vi "host.vi"() -> ()   [LabVIEW 2020]
uses:
  <vilib>/rvi/interface/nirviOpenFPGA/nirviOpenFPGA.xnode
  <vilib>/rvi/interface/nirviCloseFPGA/nirviCloseFPGA.xnode
  <vilib>/rvi/interface/nirviMethod/nirviMethod.xnode
  <vilib>/FPGAPlugInAG/Dynamic/niLvFpga_Run_Dynamic.vi
  <vilib>/rvi/errors/niLvFpgaMergeErrorWithErrorCode.vi
  <vilib>/Analysis/NI_AALBase.lvlib
  <vilib>/Analysis/baseanly.llb/Real A x B.vi
  <vilib>/Analysis/baseanly.llb/Mean (DBL).vi
  <vilib>/Analysis/NI_AALPro.lvlib
  <vilib>/Analysis/7linalg.llb/Real Cholesky Factorization.vi
  <vilib>/Analysis/7linalg.llb/Real Transpose Matrix.vi
  <vilib>/Analysis/baseanly.llb/Real Inverse Matrix.vi
  <vilib>/Analysis/7linalg.llb/Real Eigenvalues and Vectors.vi
  <vilib>/rvi/interface/nirviReadWriteControl/nirviReadWriteControl.xnode
  <vilib>/FPGAPlugInAG/Dynamic/niLvFpga_WriteFifo_Dynamic.vi
  NiFpgaLv.dll
  <vilib>/Utility/error.llb/Error Cluster From Error Code.vi
  <vilib>/rvi/interface/Simulation/niFpgaSimulationCallBeginRW.vi
  <vilib>/rvi/errors/niLvFpgaAdjustHostInterfaceError.vi
  <vilib>/FPGAPlugInAG/Dynamic/niLvFpga_ReadFifo_Dynamic.vi
  <vilib>/FPGAPlugInAG/Dynamic/niLvFpga_Close_Dynamic.vi
  FPGA Bitfiles/labviewfpgacheck_FPGATarget2_target_3W1cPbM74FU.lvbitx
  target.vi
  <vilib>/FPGAPlugInAG/PXIe-5763 (KU060)/niLvFpga_Open_PXIe-5763 (KU060).vi
  <vilib>/rvi/interface/common/dynamic/niFpgaDynamicAddResources.vi
panel:
  out "time (ms)":dbl
  out "tick count":u32
  out "LabVIEW eigvals":dbl[](array[numeric])
  out "FPGA Jacobi eigenvalue":sgl[](array[numeric])
  out "percent error":dbl
  out "A":sgl[][](array[numeric])
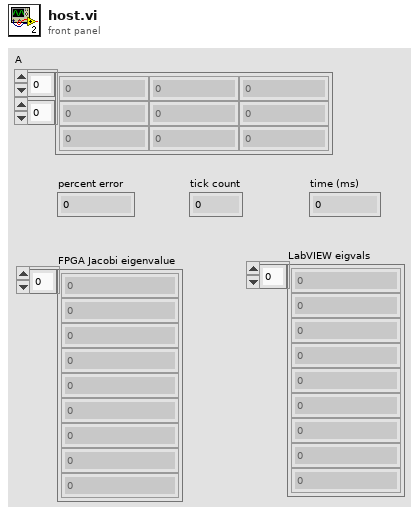
[diagram p1: front panel]
types:
  T1 = typedef "NI_Matrix.lvlib/RealMatrix.ctl" = dbl[][]
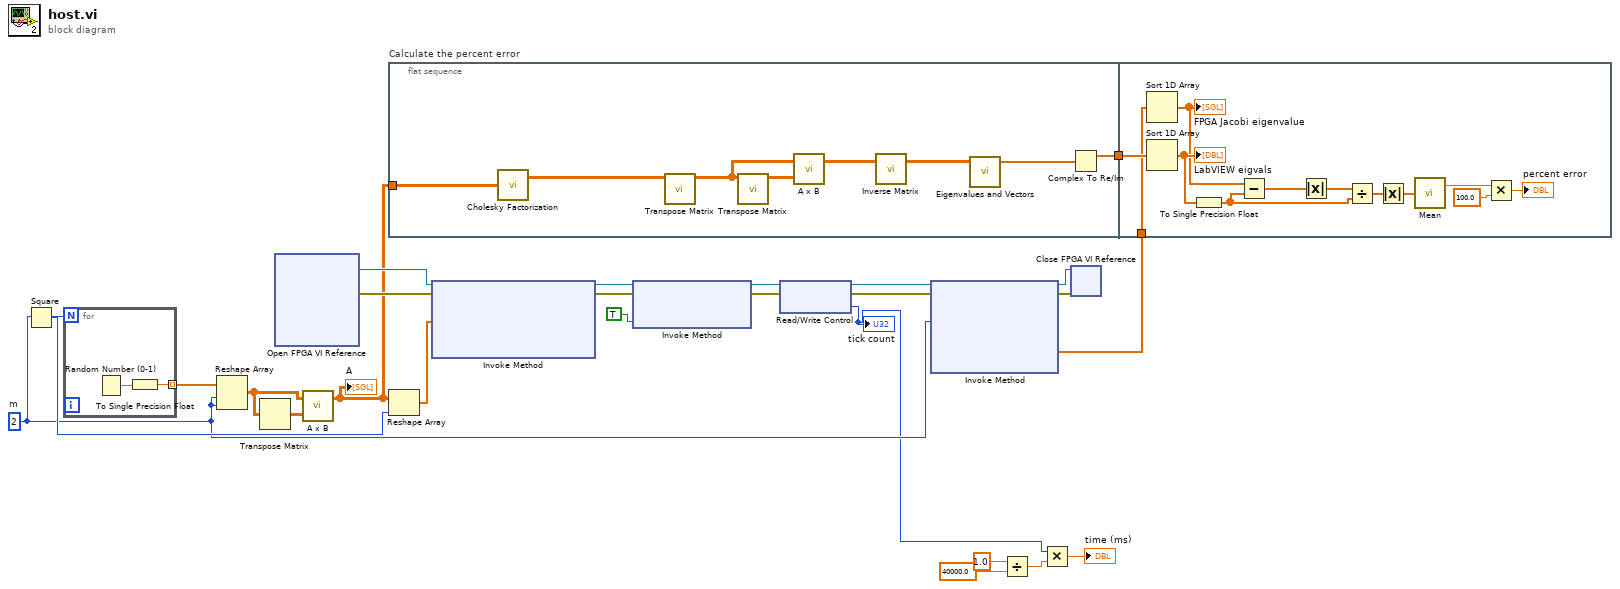
[diagram p0: block diagram]
diagram:
  w13 = 2  # m
  n1 = Square(x=w13) -> (x^2=w14:i32)
  n2 = for {
    N: w14 -> [_]
    tunnel: [w26] -> w17 mode=indexing
    n3 = Random Number (0-1)() -> (number: 0 to 1=w27:dbl)
    n4 = To Single Precision Float(number=w27) -> (single precision float=w26:sgl)
  }
  n5 = Reshape Array(w17, w13, w13) -> (w15:sgl[][])
  n6 = Transpose Matrix(1:w15) -> (0:w16:dbl[][])
  n7 = xnode "Open FPGA VI Reference"() -> ("FPGA VI Reference Out"=w24:refnum<k20>, "error out"=w23:errorcluster)  [unwired: 2 in]
  n8 = call-poly <vilib>:"A x B.vi"("B"=w16, "A"=w15) -> ("A x B"=w11:T1)  [unwired: 1 out]
  "A" <- w11
  n9 = flat-sequence "Calculate the percent error" {
    tunnel: [w28] -> w12
    tunnel: w11 -> [w29]
    tunnel: w12 -> [w47]
    tunnel: w10 -> [w36]
    frame #0 {
      n10 = call-poly <vilib>:"Cholesky Factorization.vi"("A"=w29) -> ("Cholesky"=w30:T1)  [unwired: 1 out]
      n11 = call-poly <vilib>:"Transpose Matrix.vi"("Input Matrix"=w30) -> ("Matrix Transpose"=w32:T1)  [unwired: 9 in, 1 out]
      n12 = call-poly <vilib>:"Transpose Matrix.vi"("Input Matrix"=w32) -> ("Matrix Transpose"=w31:T1)  [unwired: 9 in, 1 out]
      n13 = call-poly <vilib>:"A x B.vi"("B"=w31, "A"=w32) -> ("A x B"=w33:T1)  [unwired: 1 out]
      n14 = call-poly <vilib>:"Inverse Matrix.vi"("Input Matrix"=w33) -> ("Inverse Matrix"=w34:T1)  [unwired: 1 in, 1 out]
      n15 = call-poly <vilib>:"Eigenvalues and Vectors.vi"("Input Matrix"=w34) -> ("Eigenvalues"=w35:cdb[])  [unwired: 2 in, 2 out]
      n16 = Complex To Re/Im(x + iy=w35) -> (x=w28:dbl[])  [unwired: 1 out]
    }
    frame #1 {
      n17 = Sort 1D Array(array=w36) -> (sorted array=w45:sgl[])
      "FPGA Jacobi eigenvalue" <- w45
      n18 = Sort 1D Array(array=w47) -> (sorted array=w46:dbl[])
      "LabVIEW eigvals" <- w46
      n19 = To Single Precision Float(number=w46) -> (single precision float=w42:sgl[])
      n20 = Subtract(x=w45, y=w42) -> (x-y=w44:sgl[])
      n21 = Absolute Value(x=w44) -> (abs(x)=w43:sgl[])
      n22 = Divide(x=w43, y=w42) -> (x/y=w41:sgl[])
      n23 = Absolute Value(x=w41) -> (abs(x)=w40:sgl[])
      n24 = call-poly <vilib>:"Mean.vi"("X"=w40) -> ("mean"=w39:dbl)  [unwired: 1 out]
      n25 = Multiply(x=w39, y=100.0) -> (x*y=→"percent error":dbl)
    }
  }
  n26 = Reshape Array(w11, w14) -> (w20:dbl[])
  n27 = xnode "Invoke Method"("FPGA VI Reference In"=w24, "error in"=w23, "Data"=w20) -> ("FPGA VI Reference Out"=w19:refnum<k20>, "error out"=w18:errorcluster)  [unwired: 1 in, 1 out]
  n28 = xnode "Invoke Method"("FPGA VI Reference In"=w19, "error in"=w18, "Wait Until Done (F)"=TRUE) -> ("FPGA VI Reference Out"=w9:refnum<k20>, "error out"=w8:errorcluster)
  n29 = xnode "Read/Write Control"("FPGA VI Reference In"=w9, "error in"=w8) -> ("FPGA VI Reference Out"=w7:refnum<k20>, "error out"=w6:errorcluster, "tick count"=w2:u32)
  "tick count" <- w2
  n30 = xnode "Invoke Method"("FPGA VI Reference In"=w7, "error in"=w6, "Number of Elements"=w13) -> ("FPGA VI Reference Out"=w22:refnum<k20>, "error out"=w21:errorcluster, "Data"=w10:sgl[])  [unwired: 1 in, 1 out]
  n31 = Divide(x=1.0, y=40000.0) -> (x/y=w3:dbl)
  n32 = Multiply(x=w2, y=w3) -> (x*y=→"time (ms)":dbl)
  n33 = xnode "Close FPGA VI Reference"("FPGA VI Reference In"=w22, "error in"=w21) -> ()  [unwired: 1 out]
